vi "Get Payload.vi"(8 "error in (no error)":errorcluster, 11 "ProtobufResponse in":refnum<class "ProtobufResponse.lvclass">) -> (0 "error out":errorcluster, 2 "Payload":string, 3 "ProtobufResponse out":refnum<class "ProtobufResponse.lvclass">)   [LabVIEW 2020, in "Vecto.lvlib" / "ProtobufResponse.lvclass"]
uses:
  ProtobufResponse.lvclass
  ProtobufResponse.lvclass/ProtobufResponse.ctl
  <vilib>/IlluminatedG/IG Protoc/LV-Proto/Message/Message.lvclass
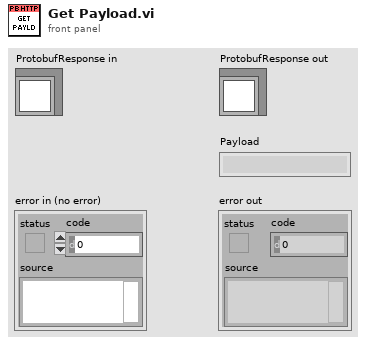
[diagram p1: front panel]
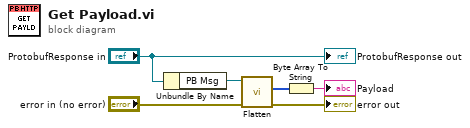
[diagram p0: block diagram]
diagram:
  n1 = Unbundle By Name("ProtobufResponse in") -> ("PB Msg"=w5:refnum<class "Message.lvclass">)
  n2 = call-dynamic "Flatten.vi"("error in (no error)"="error in (no error)", "Message in"=w5) -> ("error out"=→"error out":errorcluster, "Buffer"=w2:u8[])  [unwired: 7 in, 1 out]
  n3 = Byte Array To String(unsigned byte array=w2) -> (string=→"Payload":string)
  "ProtobufResponse out" <- "ProtobufResponse in"
